vi "LIN Trans Frame.vi"(3 "error in (no error)":errorcluster, 4 "Hex and Dec":bool, 5 "data IN":T1[](array[typedef]) {"event ID" format="%x"; "payload" format="%x"; "timestamp" format="%<%.7X\n%x>T"; "type" items=["LIN Data"=64, "LIN Bus Error"=65, "LIN No Response"=66, "Delay"=224, "Log Trigger"=225, "Start Trigger"=226]; "identifier" format="%x"}) -> (0 "error OUT":errorcluster, 1 "Data Byte":string[](array[string]), 2 "Array OUT":string[][](array[string]))   [LabVIEW 2018]
uses:
  <vilib>/xnet/xnet.llb/XNET Frame LIN.ctl
  <vilib>/xnet/xnet.llb/XNET Frame Type LIN.ctl
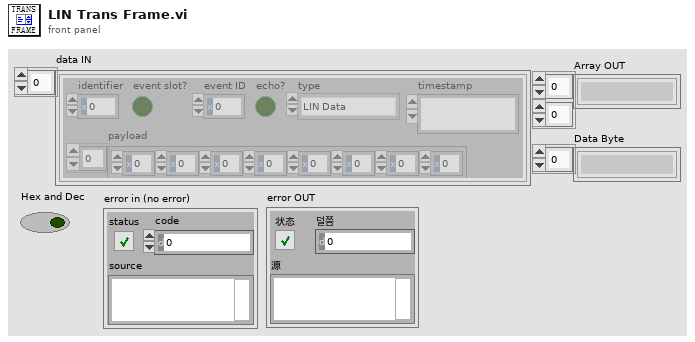
[diagram p1: front panel]
types:
  T1 = typedef "XNET Frame LIN.ctl" = cluster{"timestamp":timestamp, "payload":u8[], "identifier":u32, "type":T2, "event ID":u8, "event slot?":bool, "echo?":bool}
  T2 = typedef "XNET Frame Type LIN.ctl" = u8
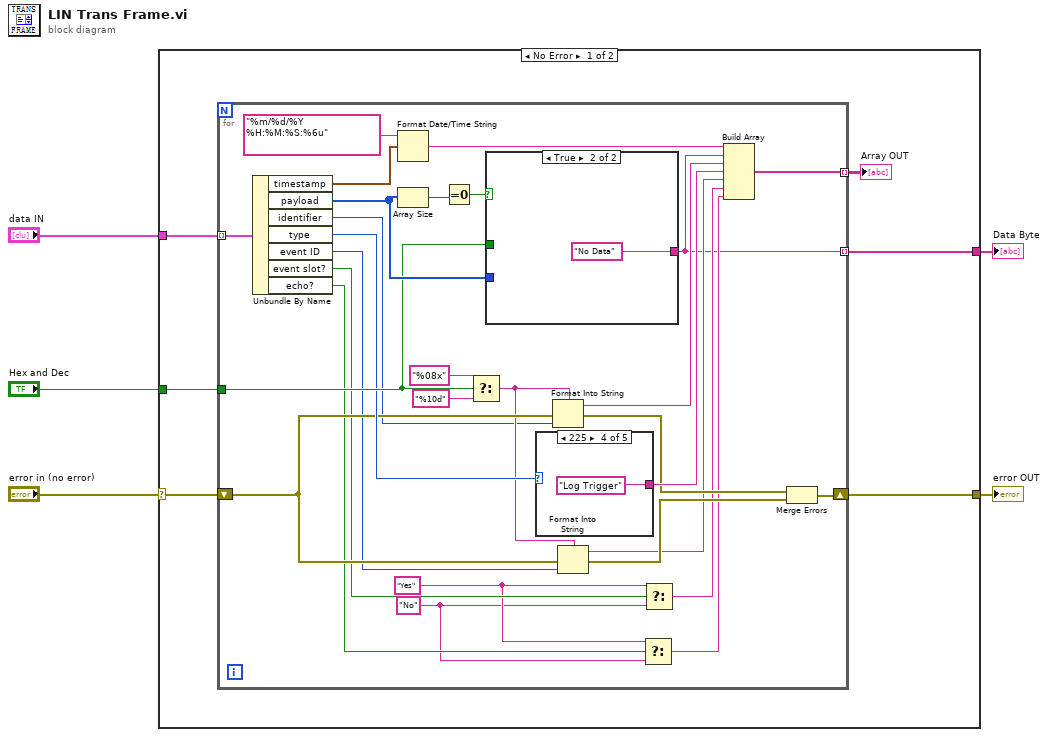
[diagram p0: block diagram]
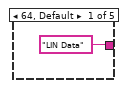
[diagram p2: hidden frame]
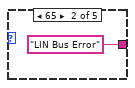
[diagram p3: hidden frame]
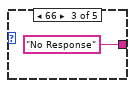
[diagram p4: hidden frame]
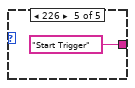
[diagram p5: hidden frame]
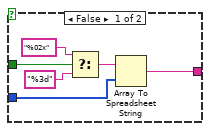
[diagram p6: hidden frame]
diagram:
  n1 = case shown="No Error" "error in (no error)" {
    selector: "error in (no error)" -> [w9 w53]
    tunnel: "Hex and Dec" -> [w10 _]
    tunnel: "data IN" -> [w11 _]
    tunnel: [w7 _] -> w2
    tunnel: [w6 w53] -> w1
    frame No Error {
      n2 = for {
        tunnel: w11 -> [w40] mode=indexing
        tunnel: w10 -> [w33]
        shift-right: [w27] -> w6
        shift-left: w9 -> [w25]
        tunnel: [w15] -> w8 mode=indexing
        tunnel: [w14] -> w7 mode=indexing
        w18 = "No"
        w19 = "Yes"
        n3 = Unbundle By Name(w40) -> ("timestamp"=w38:timestamp, "payload"=w35:u8[], "identifier"=w13:u32, "type"=w29:T2, "event ID"=w12:u8, "event slot?"=w21:bool, "echo?"=w20:bool)
        n4 = Format Date/Time String(time format string (%c)="%m/%d/%Y %H:%M:%S:%6u", seconds (now)=w38) -> (date/time string=w34:string)  [unwired: 1 in]
        n5 = Array Size(array=w35) -> (size(s)=w37:i32)
        n6 = Equal To 0?(x=w37) -> (x = 0?=w36:bool)
        n7 = Select(t="%08x", s=w33, f="%10d") -> (s? t:f=w23:string)
        n8 = case shown="True" w36 {
          tunnel: w33 -> [w51 _]
          tunnel: w35 -> [w47 _]
          tunnel: [w46 "No Data"] -> w14
          frame False {
            n9 = Select(t="%02x", s=w51, f="%3d") -> (s? t:f=w48:string)
            n10 = Array To Spreadsheet String(array=w47, 3:w48) -> (spreadsheet string=w46:string)  [unwired: 1 in]
          }
          frame True {
          }
        }
        n11 = case shown="225" w29 {
          tunnel: ["LIN Data" "LIN Bus Error" "No Response" "Log Trigger" "Start Trigger"] -> w28
          frame 64, Default {
          }
          frame 65 {
          }
          frame 66 {
          }
          frame 225 {
          }
          frame 226 {
          }
        }
        n12 = Format Into String(format string=w23, error in=w25, w13) -> (resulting string=w30:string, error out=w26:errorcluster)  [unwired: 1 in]
        n13 = Format Into String(format string=w23, error in=w25, w12) -> (resulting string=w22:string, error out=w24:errorcluster)  [unwired: 1 in]
        n14 = Select(t=w19, s=w20, f=w18) -> (s? t:f=w16:string)
        n15 = Select(t=w19, s=w21, f=w18) -> (s? t:f=w17:string)
        n16 = Build Array(w34, w14, w30, w28, w22, w17, w16) -> (w15:string[])
        n17 = Merge Errors(w26, w24) -> (w27:errorcluster)
      }
      "Array OUT" <- w8
    }
    frame Error {
    }
  }
  "Data Byte" <- w2
  "error OUT" <- w1
